vi "Get Valid Properties.vi"(0 "Filter in":refnum<class "Filter.lvclass">, 11 "error in (no error)":errorcluster) -> (4 "Filter out":refnum<class "Filter.lvclass">, 8 "Properties":string[](array[string]), 15 "error out":errorcluster)   [LabVIEW 2020, in "Filter.lvclass"]
uses:
  Filter.lvclass
  Filter.lvclass/Filter.ctl
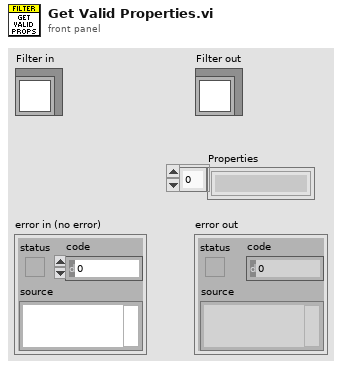
[diagram p1: front panel]
types:
  T1 = typedef "Filter.lvclass/Shape.ctl" = enum16{"OFF", "Lowpass", "Highpass", "Bandpass", "Bandstop"}
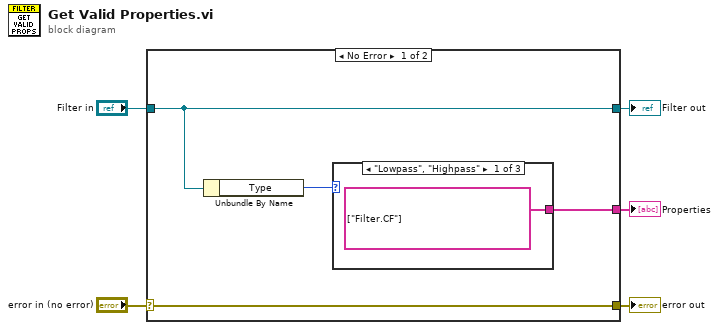
[diagram p0: block diagram]
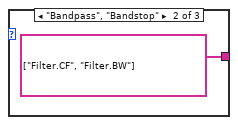
[diagram p2: hidden frame]
diagram:
  n1 = case shown="No Error" "error in (no error)" {
    selector: "error in (no error)" -> [w9 w13]
    tunnel: [w9 w13] -> w4
    tunnel: [w8 w12] -> w2
    tunnel: "Filter in" -> [w8 w12]
    tunnel: [w6 _] -> w1
    frame No Error {
      n2 = Unbundle By Name(w8) -> ("Type"=w7:T1)
      n3 = case shown="\"Lowpass\", \"Highpass\"" w7 {
        tunnel: [string[] ["Filter.CF"] string[] ["Filter.CF", "Filter.BW"] _] -> w6
        frame "Lowpass", "Highpass" {
        }
        frame "Bandpass", "Bandstop" {
        }
        frame "OFF", Default {
        }
      }
    }
    frame Error {
    }
  }
  "error out" <- w4
  "Filter out" <- w2
  "Properties" <- w1
